vi "DMA.Configure.vi"(7 "Transfer Direction":enum16{"Write", "Read"}(ring), 8 "error in (no error)":errorcluster, 10 "DMA Transfer Spec":T1 {"Block Descriptors"."next descriptor ptr" format="%08x"; "Block Descriptors"."data size" format="%08x"; "Block Descriptors"."data ptr (upper)" format="%08x"; "Block Descriptors"."data ptr (lower)" format="%08x"; "Block Descriptors"."descriptor ptr (aligned)" format="%08x"; "Block Descriptors"."descriptor size" format="%08x"; "Block Descriptors"."descriptor ptr (VISA)" format="%08x"; "RFM Address" format="%08x"}, 11 "GE 5565PIORC":refnum<class "GE 5565PIORC.lvclass">) -> (0 "error out":errorcluster, 2 "DMA Transfer Spec out":T1 {"Block Descriptors"."next descriptor ptr" format="%08x"; "Block Descriptors"."data size" format="%08x"; "Block Descriptors"."data ptr (upper)" format="%08x"; "Block Descriptors"."data ptr (lower)" format="%08x"; "Block Descriptors"."descriptor ptr (aligned)" format="%08x"; "Block Descriptors"."descriptor size" format="%08x"; "Block Descriptors"."descriptor ptr (VISA)" format="%08x"; "RFM Address" format="%08x"}, 3 "GE 5565PIORC out":refnum<class "GE 5565PIORC.lvclass">)   [LabVIEW 2016, in "GE 5565PIORC.lvclass"]
uses:
  GE 5565PIORC.lvclass
  Controls/DMA Transfer Spec.ctl
  Controls/DMA Block Descriptor.ctl
  GE 5565PIORC.lvclass/GE 5565PIORC.ctl
  Registers/Local Configuration.Get Register Offset.vi
  Binary Operations/Set Bits.vi
  Binary Operations/Set Bits U32.vi
  Binary Operations/Get Bits.vi
  Binary Operations/Get Bits U32.vi
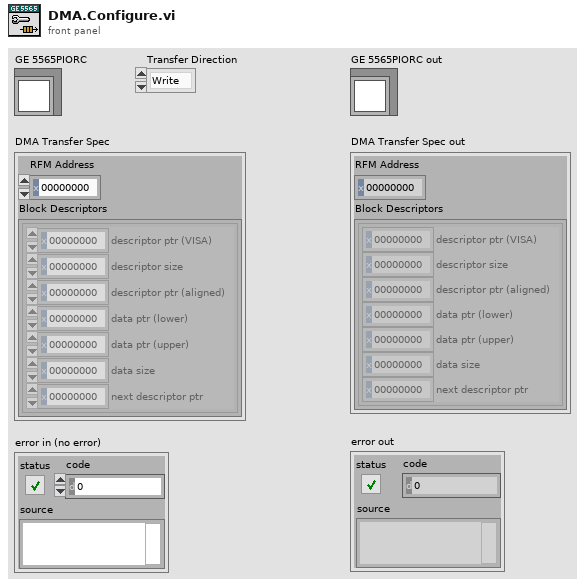
[diagram p1: front panel]
types:
  T1 = typedef "GE 5565PIORC.lvclass/DMA Transfer Spec.ctl" = cluster{"RFM Address":u32, "Block Descriptors":T2[]}
  T2 = typedef "GE 5565PIORC.lvclass/DMA Block Descriptor.ctl" = cluster{"descriptor ptr (VISA)":u32, "descriptor size":u32, "descriptor ptr (aligned)":u32, "data ptr (lower)":u32, "data ptr (upper)":u32, "data size":u32, "next descriptor ptr":u32}
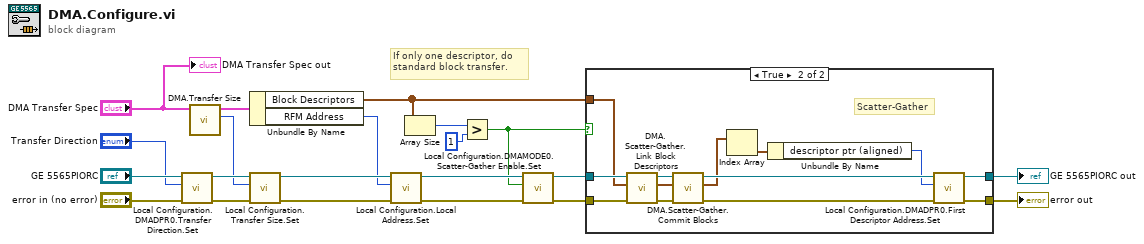
[diagram p0: block diagram]
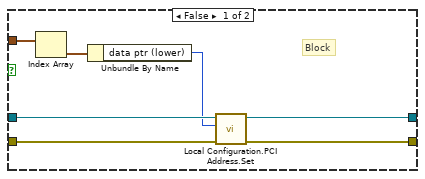
[diagram p2: hidden frame]
diagram:
  # "If only one descriptor, do standard block transfer."
  n1 = call "Local Configuration.DMADPR0.Transfer Direction.Set.vi"("error in (no error)"="error in (no error)", "Transfer Direction"="Transfer Direction", "GE 5565PIORC"="GE 5565PIORC") -> ("error out"=w10:errorcluster, "GE 5565PIORC out"=w11:refnum<class "GE 5565PIORC.lvclass">)  [unwired: 7 in]
  n2 = call "DMA.Transfer Size.vi"("DMA Transfer Spec"="DMA Transfer Spec") -> ("Transfer Size (bytes)"=w8:u32, "DMA Transfer Spec out"=w16:T1)  [unwired: 9 in]
  n3 = Unbundle By Name(w16) -> ("Block Descriptors"=w19:T2[], "RFM Address"=w13:u32)
  n4 = call "Local Configuration.Transfer Size.Set.vi"("error in (no error)"=w10, "Transfer Size"=w8, "GE 5565PIORC"=w11) -> ("error out"=w14:errorcluster, "GE 5565PIORC out"=w15:refnum<class "GE 5565PIORC.lvclass">)  [unwired: 7 in]
  n5 = call "Local Configuration.Local Address.Set.vi"("error in (no error)"=w14, "Local Address"=w13, "GE 5565PIORC"=w15) -> ("error out"=w6:errorcluster, "GE 5565PIORC out"=w5:refnum<class "GE 5565PIORC.lvclass">)  [unwired: 7 in]
  n6 = Array Size(array=w19) -> (size(s)=w18:i32)
  n7 = Greater?(x=w18, y=1) -> (0:w4:bool)
  n8 = call "Local Configuration.DMAMODE0.Scatter-Gather Enable.Set.vi"("error in (no error)"=w6, "Enable Scatter-Gather DMA?"=w4, "GE 5565PIORC"=w5) -> ("error out"=w2:errorcluster, "GE 5565PIORC out"=w3:refnum<class "GE 5565PIORC.lvclass">)  [unwired: 7 in]
  n9 = case shown="True" w4 {
    tunnel: [w22 w33] -> w21
    tunnel: [w23 w34] -> w20
    tunnel: w2 -> [w27 w38]
    tunnel: w3 -> [w28 w37]
    tunnel: w19 -> [w26 w35]
    frame False {
      # "Block"
      n10 = Index Array(array=w26) -> (element=w25:T2)  [unwired: 1 in]
      n11 = Unbundle By Name(w25) -> ("data ptr (lower)"=w24:u32)
      n12 = call "Local Configuration.PCI Address.Set.vi"("error in (no error)"=w27, "PCI Address"=w24, "GE 5565PIORC"=w28) -> ("error out"=w22:errorcluster, "GE 5565PIORC out"=w23:refnum<class "GE 5565PIORC.lvclass">)  [unwired: 7 in]
    }
    frame True {
      # "Scatter-Gather"
      n13 = call "DMA.Scatter-Gather.Link Block Descriptors.vi"("error in (no error)"=w38, "Block Descriptors"=w35, "GE 5565PIORC in"=w37) -> ("error out"=w36:errorcluster, "Block Descriptors out"=w40:T2[], "GE 5565PIORC out"=w39:refnum<class "GE 5565PIORC.lvclass">)  [unwired: 6 in]
      n14 = call "DMA.Scatter-Gather.Commit Blocks.vi"("error in (no error)"=w36, "Block Descriptors"=w40, "GE 5565PIORC in"=w39) -> ("error out"=w31:errorcluster, "Block Descriptors out"=w30:T2[], "GE 5565PIORC out"=w32:refnum<class "GE 5565PIORC.lvclass">)  [unwired: 6 in]
      n15 = Index Array(array=w30) -> (element=w41:T2)  [unwired: 1 in]
      n16 = Unbundle By Name(w41) -> ("descriptor ptr (aligned)"=w29:u32)
      n17 = call "Local Configuration.DMADPR0.First Descriptor Address.Set.vi"("error in (no error)"=w31, "First Descriptor Address"=w29, "GE 5565PIORC"=w32) -> ("error out"=w33:errorcluster, "GE 5565PIORC out"=w34:refnum<class "GE 5565PIORC.lvclass">)  [unwired: 7 in]
    }
  }
  "error out" <- w21
  "GE 5565PIORC out" <- w20
  "DMA Transfer Spec out" <- "DMA Transfer Spec"
